vi "MoveShip.vi"(0 "MainCluster_IN":T11, 1 "Direction":string) -> (2 "MainCluster _OUT":T11)   [LabVIEW 2022 SP3]
uses:
  InitCluster.ctl
  CharacterCluster.ctl
  <vilib>/picture/picture.llb/imagedata.ctl
  ShotInitCluster.ctl
  <vilib>/Utility/miscctls.llb/LVPositionTypeDef.ctl
  <vilib>/Utility/miscctls.llb/LVBoundsTypeDef.ctl
  ShotCluster.ctl
  move_dir_ud.ctl
  InvaderPositionArray.ctl
  move_dir_lr.ctl
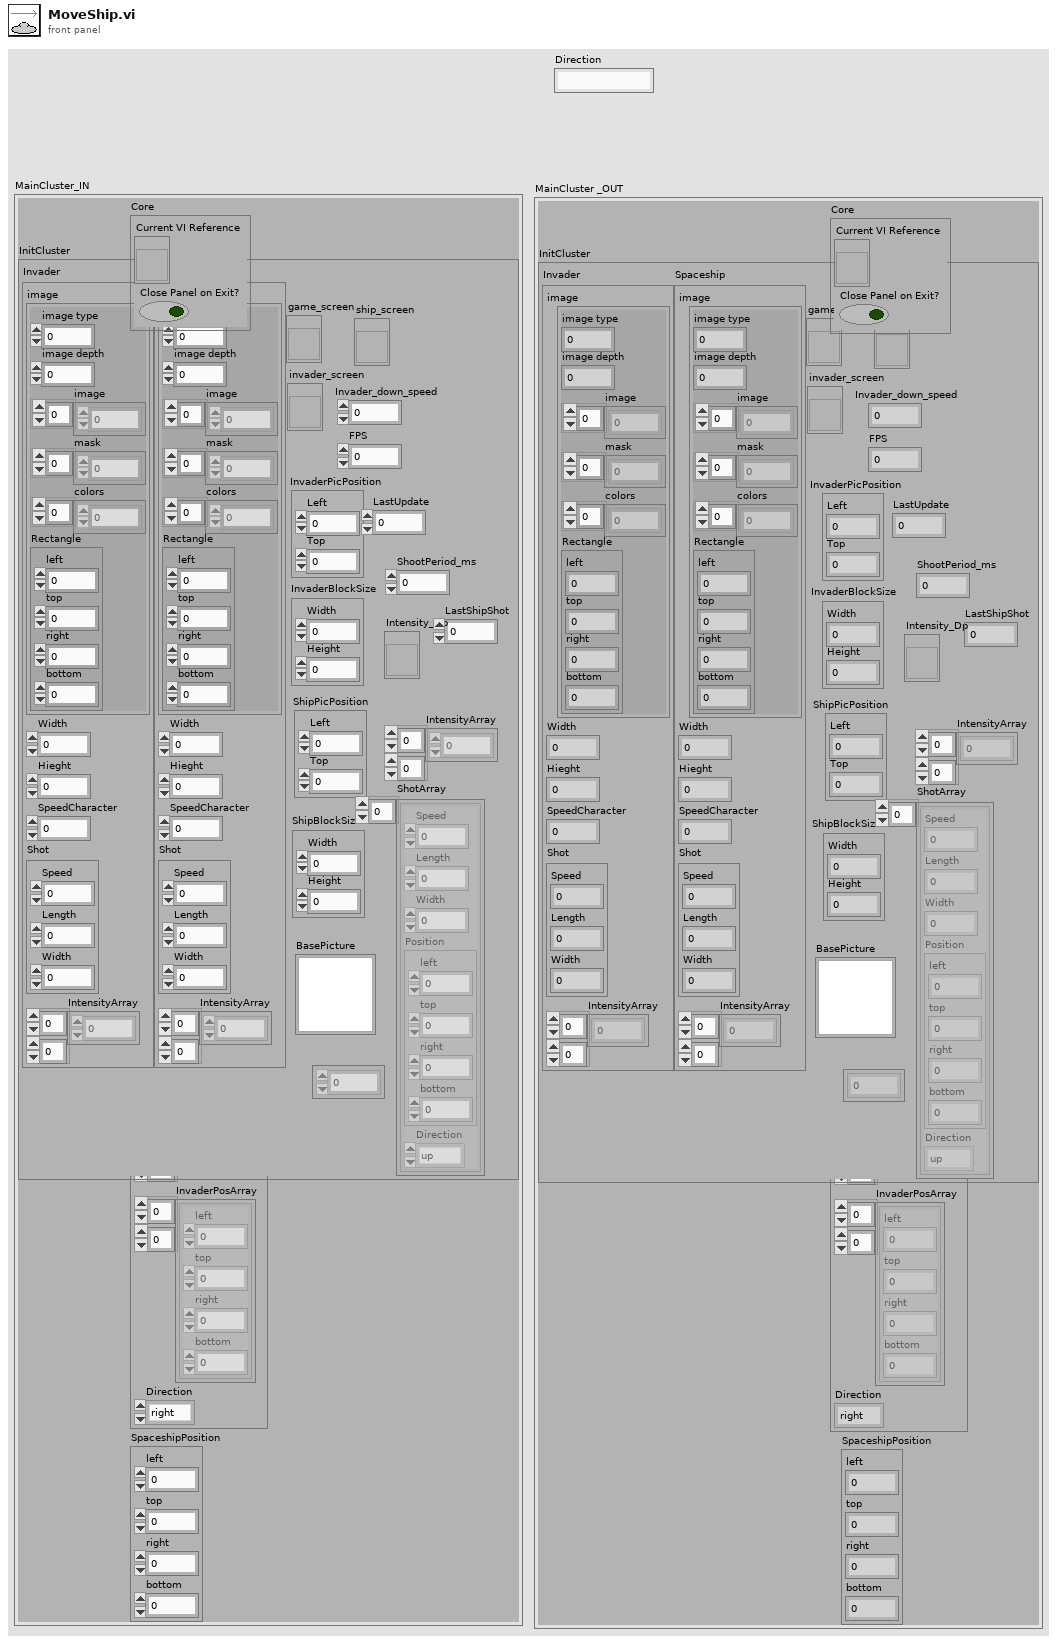
[diagram p1: front panel]
types:
  T1 = typedef "InitCluster.ctl" = cluster{"Invader":T2, "Spaceship":T2, "game_screen":refnum<vi>, "BasePicture":picture, "invader_screen":refnum<vi>, "InvaderPicPosition":T5, "Invader_down_speed":i16, "FPS":u16, "InvaderBlockSize":T6, "ship_screen":refnum<vi>, "ShipBlockSize":T6, "ShipPicPosition":T5, "LastUpdate":u32, "Intensity_Dp":refnum<vi>, "IntensityArray":u8[][], "ShotArray":T7[], "InvaderShotTimeArray":u32[], "ShootPeriod_ms":i32, "LastShipShot":u32}
  T2 = typedef "CharacterCluster.ctl" = cluster{"image":T3, "Width":u32, "Hieght":u32, "SpeedCharacter":u32, "Shot":T4, "IntensityArray":u8[][]}
  T3 = typedef "imagedata.ctl" = cluster{"image type":i32, "image depth":i32, "image":u8[], "mask":u8[], "colors":u32[], "Rectangle":cluster{"left":i16, "top":i16, "right":i16, "bottom":i16}}
  T4 = typedef "ShotInitCluster.ctl" = cluster{"Speed":u32, "Length":u32, "Width":u32}
  T5 = typedef "LVPositionTypeDef.ctl" = cluster{"Left":i32, "Top":i32}
  T6 = typedef "LVBoundsTypeDef.ctl" = cluster{"Width":u32, "Height":u32}
  T7 = typedef "ShotCluster.ctl" = cluster{"Speed":u32, "Length":u32, "Width":u32, "Position":cluster{"left":i16, "top":i16, "right":i16, "bottom":i16}, "Direction":T8}
  T8 = typedef "move_dir_ud.ctl" = enum16{"up", "down"}
  T9 = typedef "InvaderPositionArray.ctl" = cluster{"InvaderAlive":bool[][], "InvaderPosArray":cluster{"left":i16, "top":i16, "right":i16, "bottom":i16}[][], "Direction":T10}
  T10 = typedef "move_dir_lr.ctl" = enum16{"right", "left"}
  T11 = cluster{"Core":cluster{"Current VI Reference":refnum<vi>, "Close Panel on Exit?":bool}, "InitCluster":T1, "InvaderPosArray":T9, "SpaceshipPosition":cluster{"left":i16, "top":i16, "right":i16, "bottom":i16}}
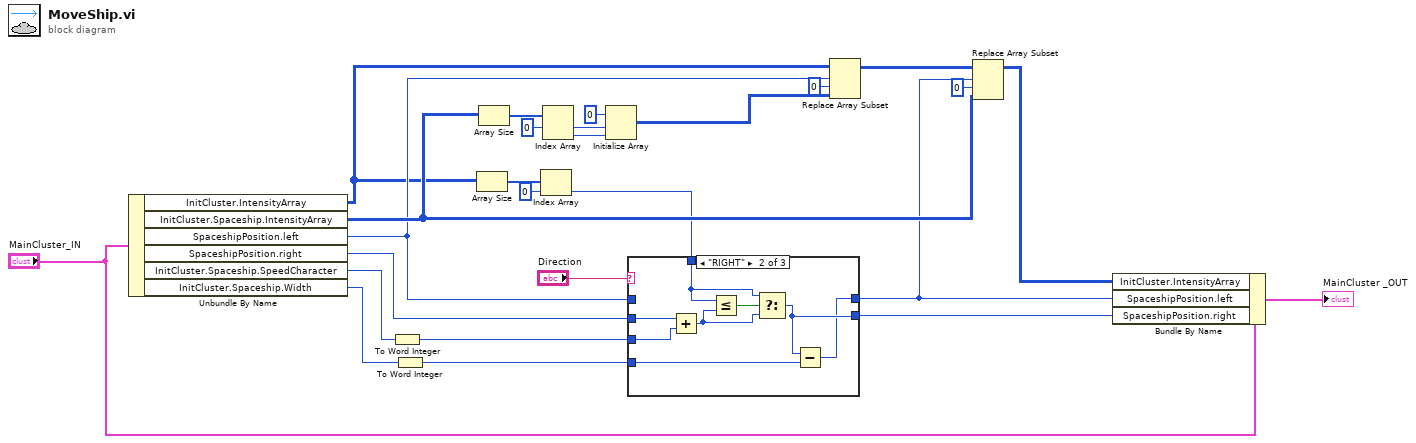
[diagram p0: block diagram]
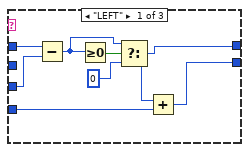
[diagram p2: hidden frame]
diagram:
  n1 = Unbundle By Name("MainCluster_IN") -> ("InitCluster.IntensityArray"=w4:u8[][], "InitCluster.Spaceship.IntensityArray"=w10:u8[][], "SpaceshipPosition.left"=w8:i16, "SpaceshipPosition.right"=w26:i16, "InitCluster.Spaceship.SpeedCharacter"=w24:u32, "InitCluster.Spaceship.Width"=w21:u32)
  n2 = To Word Integer(number=w24) -> (16bit integer=w25:i16)
  n3 = To Word Integer(number=w21) -> (16bit integer=w20:i16)
  n4 = Array Size(array=w4) -> (size(s)=w3:i32[])
  n5 = Array Size(array=w10) -> (size(s)=w16:i32[])
  n6 = Index Array(array=w3, index=0) -> (element=w1:i32)
  n7 = Index Array(array=w16, index #1=0 ("index")) -> (element #1=w6:i32, element #2=w5:i32)  [unwired: 1 in]
  n8 = Initialize Array(u8 0 ("element"), w6, w5) -> (w11:u8[][])
  n9 = case shown="\"RIGHT\"" "Direction" {
    tunnel: w8 -> [w34 _ w44]
    tunnel: w26 -> [_ w42 w43]
    tunnel: w25 -> [w33 w41 _]
    tunnel: w1 -> [_ w39 _]
    tunnel: [w27 w35 w44] -> w9
    tunnel: w20 -> [w32 w36 _]
    tunnel: [w31 w37 w43] -> w19
    frame "LEFT" {
      n10 = Subtract(x=w34, y=w33) -> (x-y=w29:i16)
      n11 = Greater Or Equal To 0?(x=w29) -> (x >= 0?=w30:bool)
      n12 = Select(t=w29, s=w30, f=i16 0) -> (s? t:f=w27:i16)
      n13 = Add(x=w27, y=w32) -> (x+y=w31:i16)
    }
    frame "RIGHT" {
      n14 = Add(x=w42, y=w41) -> (x+y=w38:i16)
      n15 = Less Or Equal?(x=w39, y=w38) -> (x <= y?=w40:bool)
      n16 = Select(t=w39, s=w40, f=w38) -> (s? t:f=w37:i32)
      n17 = Subtract(x=w37, y=w36) -> (x-y=w35:i32)
    }
    frame Default {
    }
  }
  n18 = Replace Array Subset(array=w4, new element=w11, index (row)=w8, index (col)=0 ("disabled index (col)")) -> (w13:u8[][])
  n19 = Replace Array Subset(array=w13, new element=w10, index (row)=w9, index (col)=0 ("disabled index (col)")) -> (w7:u8[][])
  n20 = Bundle By Name(cluster="MainCluster_IN", "InitCluster.IntensityArray"=w7, "SpaceshipPosition.left"=w9, "SpaceshipPosition.right"=w19) -> (→"MainCluster _OUT":T11)
